vi "Set Alarm Reason.vi"(8 "error in (no error)":errorcluster, 10 "Alarm Reason":string, 11 "Alarm in":refnum<class "Alarm.lvclass">) -> (0 "error out":errorcluster, 3 "Alarm out":refnum<class "Alarm.lvclass">)   [LabVIEW 2018, in "Alarm.lvclass"]
uses:
  Alarm.lvclass
  Alarm.lvclass/Alarm.ctl
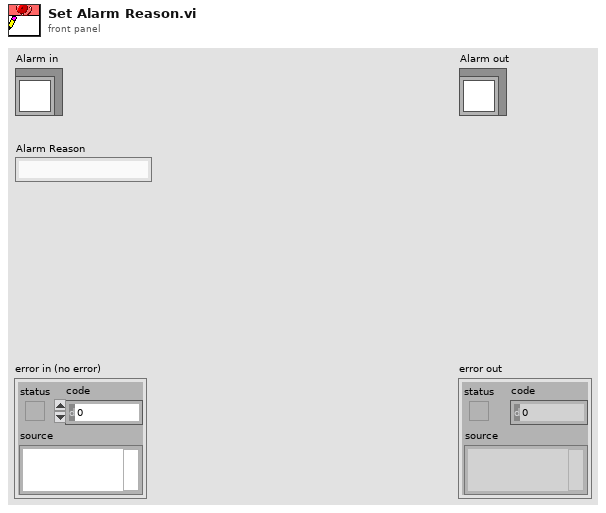
[diagram p1: front panel]
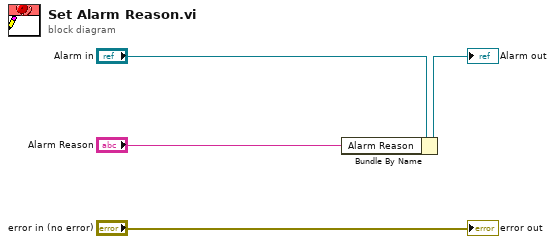
[diagram p0: block diagram]
diagram:
  n1 = Bundle By Name(cluster="Alarm in", "Alarm Reason"="Alarm Reason") -> (→"Alarm out":refnum<class "Alarm.lvclass">)
  "error out" <- "error in (no error)"
